vi "Main.vi"(8 "error in":errorcluster, 11 "Maestro Data Logg in":refnum<class "Maestro Data Logg.lvclass">) -> (0 "error out":errorcluster, 3 "Maestro Data Logg out":refnum<class "Maestro Data Logg.lvclass">)   [LabVIEW 2021, in "Maestro Data Logg.lvclass"]
doc: "The Queued Message Handler of a Worker."
uses:
  Maestro Data Logg.lvclass
  C:/Program Files (x86)/National Instruments/LabVIEW 2021/vi.lib/addons/_Workers/Library/Classes/Worker/Worker.lvclass
  Logging State.ctl
  Initialization Data.ctl
  <vilib>/addons/_Workers/Library/Classes/Message Queue/Message Queue.lvclass
  Maestro Data Logg.lvclass/Maestro Data Logg.ctl
  <vilib>/addons/_Workers/Library/Classes/Message/Enqueue Message to Self v2.vi
  <vilib>/addons/_Workers/Library/Classes/Message/Enqueue Message to Queue.vi
  <vilib>/addons/_Workers/Library/Classes/Message/Message.lvclass
  Maestro Control/Maestro Control.lvclass
  C:/Program Files (x86)/National Instruments/LabVIEW 2021/vi.lib/addons/_Workers/Library/Classes/Workers Object/Workers Object.lvclass
  C:/Users/flepetit/Desktop/Gentec-maestro-Labview/Workers/Maestro Data Logg/Maestro Data Logg.lvclass
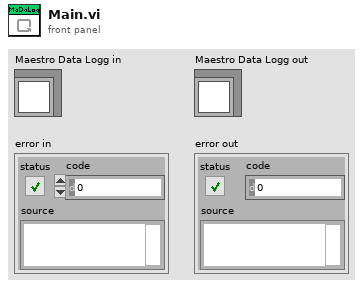
[diagram p1: front panel]
types:
  T1 = typedef "Maestro Data Logg.lvclass/Initialization Data.ctl" = cluster{"String":string, "Data Queue":refnum<queue>, "Data Notifier":refnum<notifier>, "Maestro Ctrl Queue":refnum<class "Message Queue.lvclass">, "Log File Base Path":path, "Activer les Stats":bool}
  T2 = typedef "Maestro Data Logg.lvclass/Logging State.ctl" = enum16{"Idle", "Logging"}
  T3 = enum16{"open", "open or create", "create or replace", "create", "open (read-only)"}
  T4 = cluster{"Tps(s)":dbl[], "Puiss.":dbl, "Waveform":waveform(dbl)[]}
  T5 = typedef "Workers.lvlib/Case Label.ctl" = string
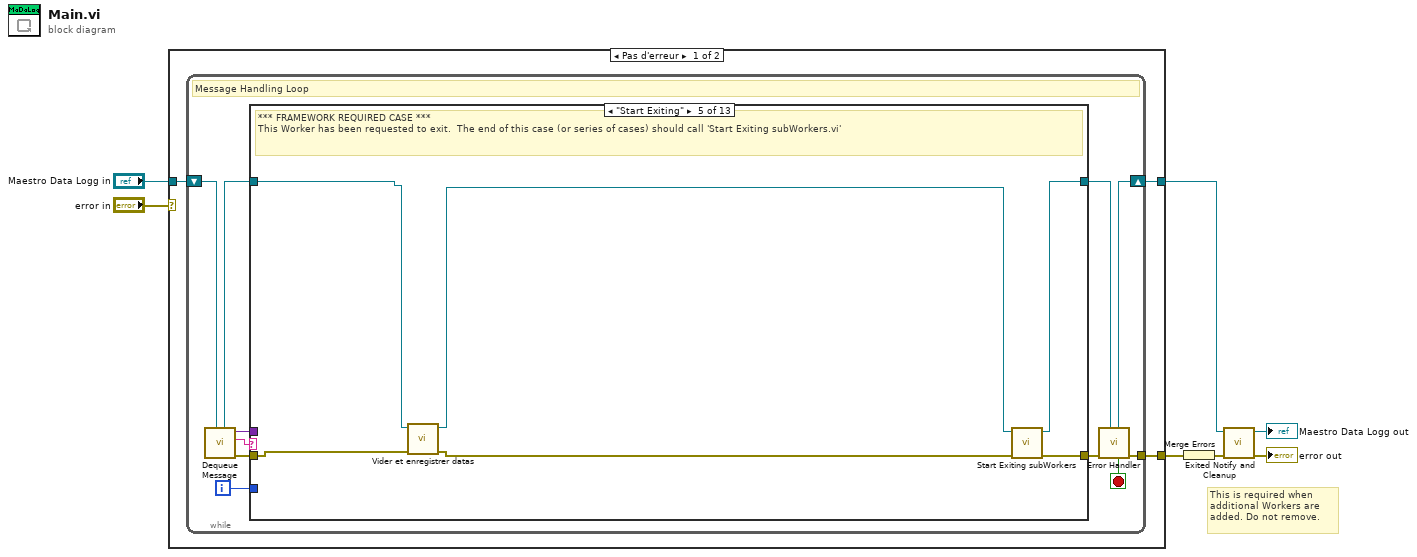
[diagram p0: block diagram]
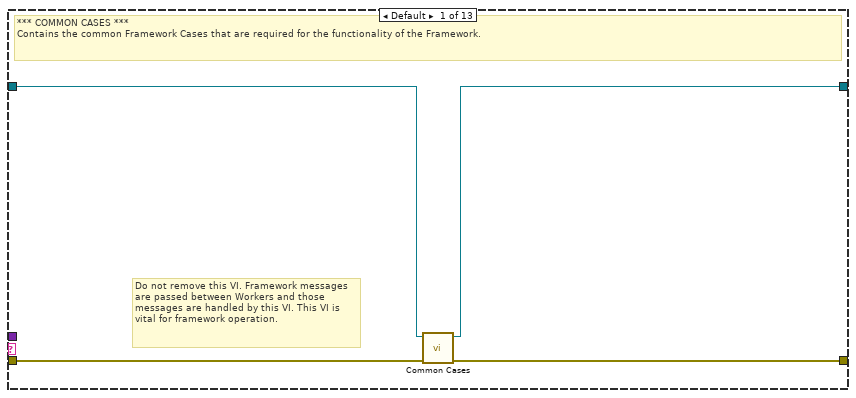
[diagram p2: hidden frame]
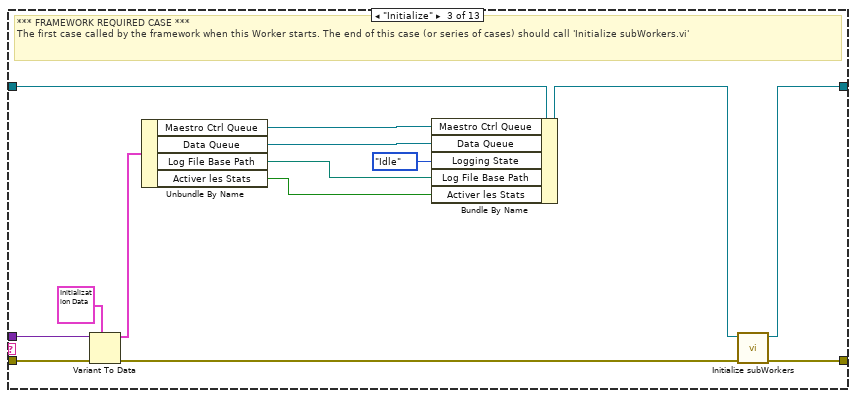
[diagram p4: hidden frame]
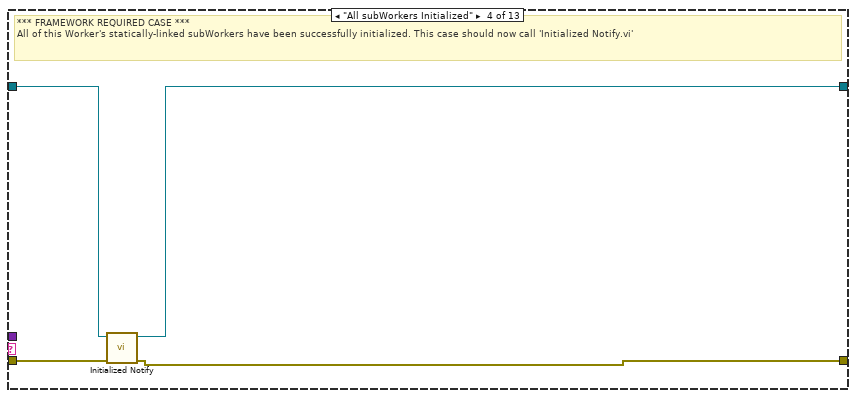
[diagram p5: hidden frame]
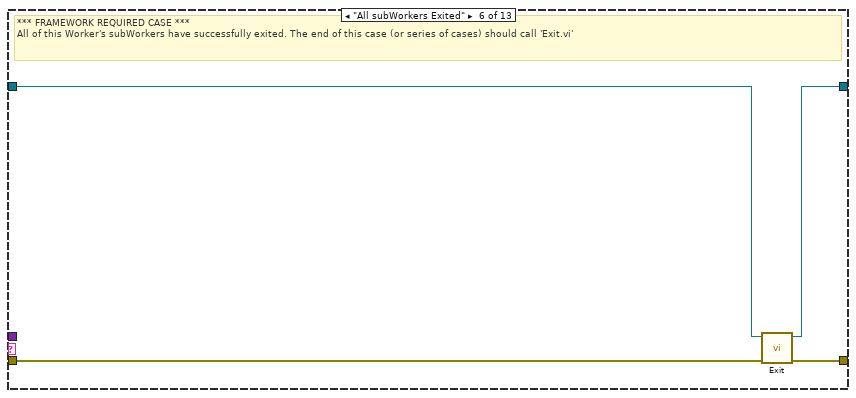
[diagram p6: hidden frame]
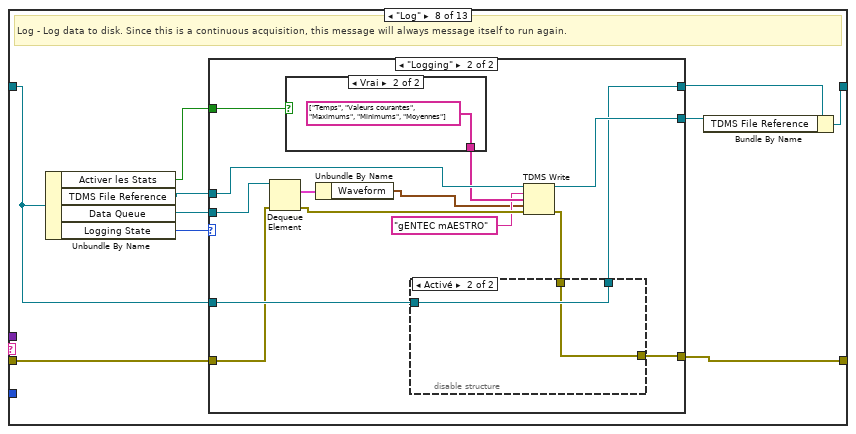
[diagram p8: hidden frame]
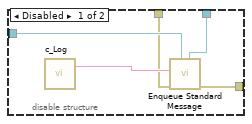
[diagram p10: hidden frame]
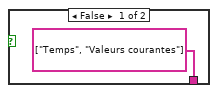
[diagram p11: hidden frame]
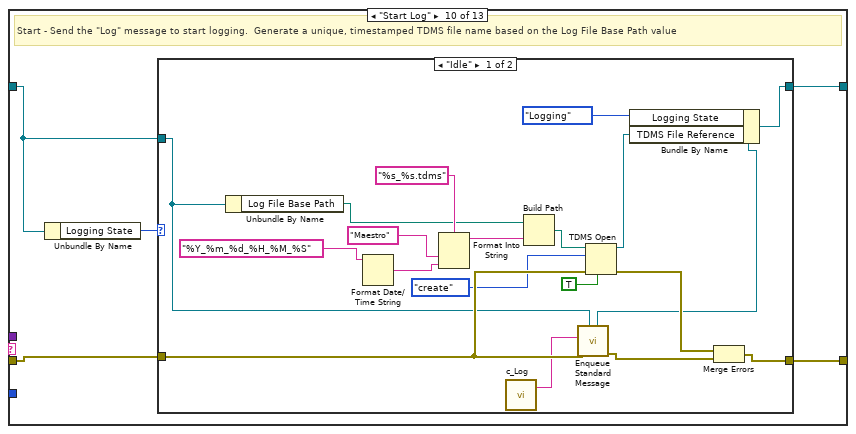
[diagram p13: hidden frame]
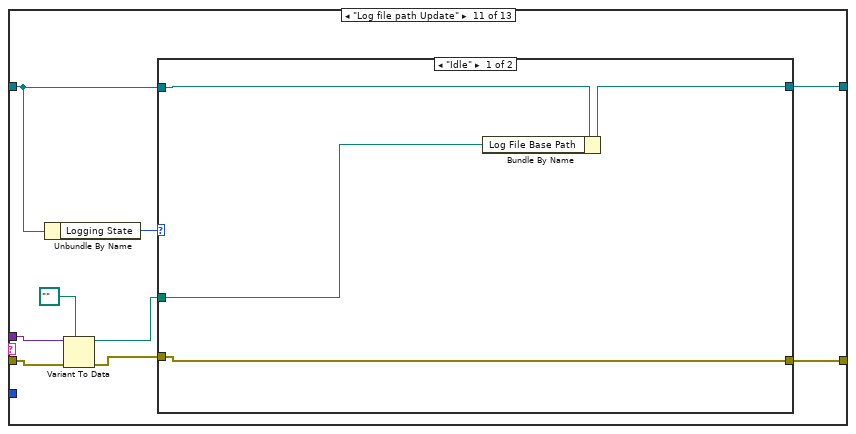
[diagram p15: hidden frame]
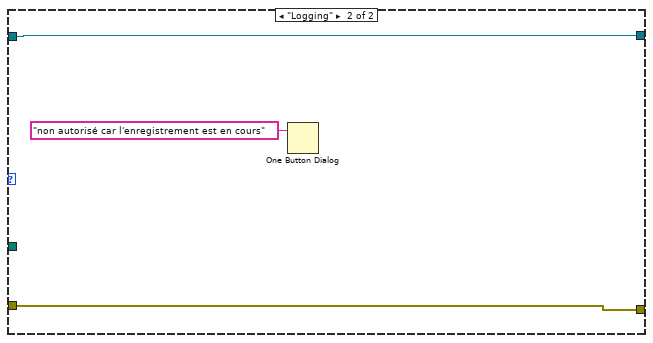
[diagram p16: hidden frame]
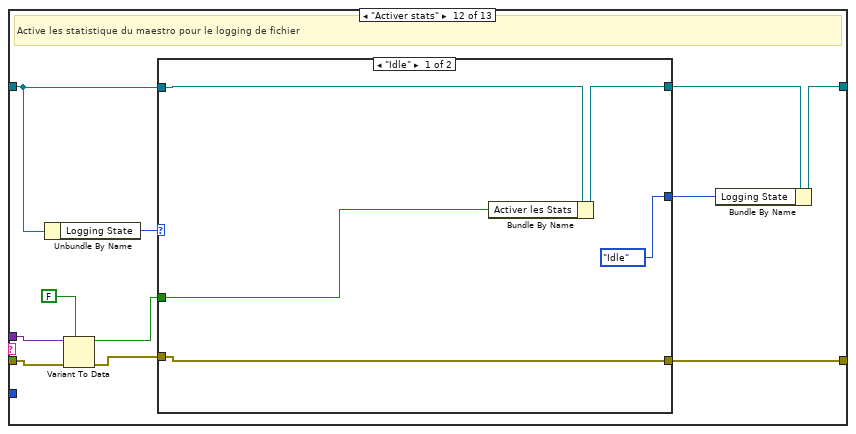
[diagram p17: hidden frame]
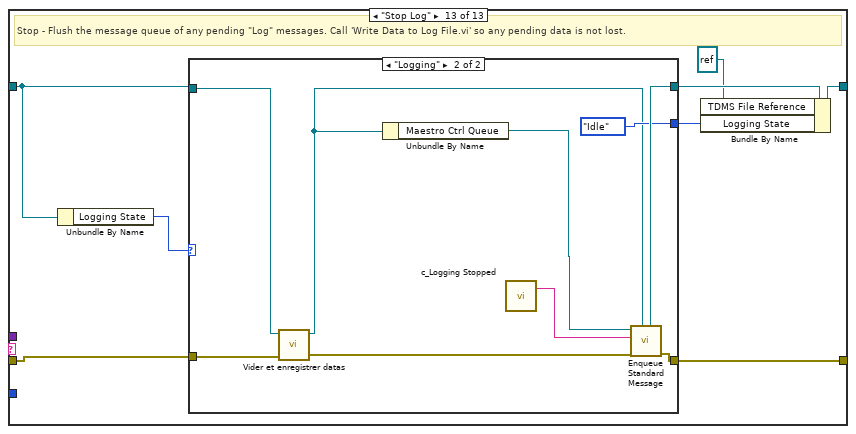
[diagram p19: hidden frame]
diagram:
  # "This is required when additional Workers are added. Do not remove."
  n1 = case shown="Pas d'erreur" "error in" {
    tunnel: "Maestro Data Logg in" -> [w8 w178]
    tunnel: [w10 w179] -> w6
    tunnel: [w9 w177] -> w7
    selector: "error in" -> [_ w180]
    frame No Error {
      n2 = while {
        shift-right: [w19] -> w9
        shift-left: w8 -> [w21]
        tunnel: [w20] -> w10
        i -> [w11]
        stop <- w12 stop-if-true
        # "Message Handling Loop"
        n3 = call-dynamic "Dequeue Message.vi"("Worker"=w21) -> ("error out"=w18:errorcluster, "Case out"=w13:string, "Data out"=w14:variant, "Worker out"=w16:refnum<class "Maestro Data Logg.lvclass">)  [unwired: 6 in, 1 out]
        n4 = case "Worker MHL Case Structure (DO NOT CHANGE LABEL NAME)" shown="\"Start Exiting\"" w13 {
          tunnel: w18 -> [w25 w26 w39 w45 w49 w55 w56 w66 w94 w96 w126 w144 w161]
          tunnel: [w24 w26 w41 w43 w51 w54 w56 w59 w94 w97 w127 w145 w162] -> w17
          tunnel: w16 -> [w23 w27 w36 w44 w47 w53 w57 w65 w95 w99 w129 w147 w163]
          tunnel: [w22 w27 w40 w42 w50 w52 w57 w60 w95 w98 w128 w139 w159] -> w15
          tunnel: w14 -> [_ _ w37 _ _ _ _ _ _ _ w124 w142 _]
          tunnel: w11 -> [_ _ _ _ _ _ _ _ _ _ _ _ _]
          frame Default {
            # "Do not remove this VI. Framework messages are passed between Workers and those messages are handled by this VI. This VI is vital for framework operation."
            # "*** COMMON CASES ***\nContains the common Framework Cases that are required for the functionality of the Framework."
            n5 = call-dynamic "Common Cases.vi"("error in"=w25, "Worker in"=w23) -> ("error out"=w24:errorcluster, "Worker out"=w22:refnum<class "Maestro Data Logg.lvclass">)  [unwired: 8 in]
          }
          frame "------ FRAMEWORK REQUIRED CASES ------" {
            # "Start of Framework Required Cases"
          }
          frame "Initialize" {
            # "*** FRAMEWORK REQUIRED CASE ***\nThe first case called by the framework when this Worker starts. The end of this case (or series of cases) should call 'Initialize subWorkers.vi'"
            n6 = Variant To Data(error in=w39, type=T1 {"String"="", "Data Queue"=refnum, "Data Notifier"=refnum, "Maestro Ctrl Queue"=refnum, "Log File Base Path"=path "", "Activer les Stats"=FALSE} ("Cluster"), Variant=w37) -> (data=w35:T1, error out=w38:errorcluster)
            n7 = Unbundle By Name(w35) -> ("Maestro Ctrl Queue"=w33:refnum<class "Message Queue.lvclass">, "Data Queue"=w32:refnum<queue>, "Log File Base Path"=w30:path, "Activer les Stats"=w29:bool)
            n8 = Bundle By Name(cluster=w36, "Maestro Ctrl Queue"=w33, "Data Queue"=w32, "Logging State"=Logging_State."Idle", "Log File Base Path"=w30, "Activer les Stats"=w29) -> (w34:refnum<class "Maestro Data Logg.lvclass">)
            n9 = call-dynamic "Initialize subWorkers.vi"("error in"=w38, "Worker"=w34) -> ("error out"=w41:errorcluster, "dup Worker out"=w40:refnum<class "Maestro Data Logg.lvclass">)  [unwired: 8 in]
          }
          frame "All subWorkers Initialized" {
            # "*** FRAMEWORK REQUIRED CASE ***\nAll of this Worker's statically-linked subWorkers have been successfully initialized. This case should now call 'Initialized Notify.vi'"
            n10 = call-dynamic "Initialized Notify.vi"("error in"=w45, "Worker"=w44) -> ("error out"=w43:errorcluster, "dup Worker out"=w42:refnum<class "Maestro Data Logg.lvclass">)  [unwired: 8 in]
          }
          frame "Start Exiting" {
            # "*** FRAMEWORK REQUIRED CASE ***\nThis Worker has been requested to exit.  The end of this case (or series of cases) should call 'Start Exiting subWorkers.vi'"
            n11 = call "Vider et enregistrer datas.vi"("error in (no error)"=w49, "Maestro Data Logg en entrée"=w47) -> ("error out"=w48:errorcluster, "Maestro Data Logg en sortie"=w46:refnum<class "Maestro Data Logg.lvclass">)  [unwired: 8 in]
            n12 = call-dynamic "Start Exiting subWorkers.vi"("error_in"=w48, "Worker"=w46) -> ("error out"=w51:errorcluster, "dup Worker out"=w50:refnum<class "Maestro Data Logg.lvclass">)  [unwired: 8 in]
          }
          frame "All subWorkers Exited" {
            # "*** FRAMEWORK REQUIRED CASE ***\nAll of this Worker's subWorkers have successfully exited. The end of this case (or series of cases) should call 'Exit.vi'"
            n13 = call-dynamic "Exit.vi"("error_in"=w55, "Worker"=w53) -> ("error out"=w54:errorcluster, "dup Worker out"=w52:refnum<class "Maestro Data Logg.lvclass">)  [unwired: 8 in]
          }
          frame "------------------Himself-------------------------" {
            # "End of Framework Required Cases"
          }
          frame "Log" {
            # "Log - Log data to disk. Since this is a continuous acquisition, this message will always message itself to run again."
            n14 = Unbundle By Name(w65) -> ("Activer les Stats"=w58:bool, "TDMS File Reference"=w63:refnum<k34>, "Data Queue"=w64:refnum<queue>, "Logging State"=w67:T2)
            n15 = case shown="\"Logging\"" w67 {
              tunnel: [w70 w74] -> w61
              tunnel: w66 -> [w69 w79]
              tunnel: [w69 w72] -> w59
              tunnel: w65 -> [w70 w84]
              tunnel: w64 -> [_ w82]
              tunnel: w63 -> [w68 w80]
              tunnel: [w68 w75] -> w62
              tunnel: w58 -> [_ w71]
              frame "Idle" {
              }
              frame "Logging" {
                n16 = Dequeue Element(queue=w82, error in (no error)=w79) -> (element=w81:T4, error out=w83:errorcluster)  [unwired: 1 in, 2 out]
                n17 = case shown="Vrai" w71 {
                  tunnel: [string[] ["Temps", "Valeurs courantes"] ("nom des voies en entrée (Sans titre)") string[] ["Temps", "Valeurs courantes", "Maximums", "Minimums", "Moyennes"] ("nom des voies en entrée (Sans titre)")] -> w78
                  frame False {
                  }
                  frame True {
                  }
                }
                n18 = Unbundle By Name(w81) -> ("Waveform"=w76:waveform(dbl)[])
                n19 = TDMS Write(0:w80, 5:"gENTEC mAESTRO" ("nom du groupe en entrée (Sans titre)"), 7:w78, 9:w76, 11:w83) -> (4:w75:refnum<k34>, 15:w73:errorcluster)  [unwired: 1 in, 2 out]
                n20 = disable-structure shown="Activé" {
                  disable-tunnel: w84 -> [w89 w91]
                  disable-tunnel: [w87 w91] -> w74
                  disable-tunnel: w73 -> [w86 w90]
                  disable-tunnel: [w85 w90] -> w72
                  frame Disabled {
                    n21 = call "c_Log.vi"() -> ("Case Label"=w88:T5)  [unwired: 1 in]
                    n22 = call-poly <vilib>:"Enqueue Standard Message.vi"("Worker"=w89, "error in"=w86, "Case Label"=w88) -> ("error out"=w85:errorcluster, "dup Worker out"=w87:refnum<class "Maestro Data Logg.lvclass">)  [unwired: 7 in]
                  }
                  frame Enabled {
                  }
                }
              }
            }
            n23 = Bundle By Name(cluster=w61, "TDMS File Reference"=w62) -> (w60:refnum<class "Maestro Data Logg.lvclass">)
          }
          frame "------------From Maestro Control--------------" {
            # "End of Framework Required Cases"
          }
          frame "Start Log" {
            # "Start - Send the \"Log\" message to start logging.  Generate a unique, timestamped TDMS file name based on the Log File Base Path value"
            n24 = Unbundle By Name(w99) -> ("Logging State"=w100:T2)
            n25 = case shown="\"Idle\"" w100 {
              tunnel: w99 -> [w108 w121]
              tunnel: [w109 w121] -> w98
              tunnel: [w115 w120] -> w97
              tunnel: w96 -> [w117 w120]
              frame "Idle" {
                n26 = Unbundle By Name(w108) -> ("Log File Base Path"=w104:path)
                n27 = Format Date/Time String(time format string (%c)="%Y_%m_%d_%H_%M_%S") -> (date/time string=w105:string)  [unwired: 2 in]
                n28 = Format Into String(format string="%s_%s.tdms", "Maestro" ("entrée 1"), w105) -> (resulting string=w119:string)  [unwired: 2 in, 1 out]
                n29 = call "c_Log.vi"() -> ("Case Label"=w101:T5)  [unwired: 1 in]
                n30 = Build Path(base path=w104, name or relative path=w119) -> (appended path=w113:path)
                n31 = call-poly <vilib>:"Enqueue Standard Message.vi"("Worker"=w108, "error in"=w117, "Case Label"=w101) -> ("error out"=w116:errorcluster, "dup Worker out"=w107:refnum<class "Maestro Data Logg.lvclass">)  [unwired: 7 in]
                n32 = TDMS Open(6:TRUE ("désactiver la bufférisation ? (V)"), 8:w117, 10:T3."create" ("operation (0:open)"), 11:w113) -> (0:w114:errorcluster, 3:w110:refnum<k34>)  [unwired: 3 in]
                n33 = Bundle By Name(cluster=w107, "Logging State"=Logging_State."Logging", "TDMS File Reference"=w110) -> (w109:refnum<class "Maestro Data Logg.lvclass">)
                n34 = Merge Errors(w114, w116) -> (w115:errorcluster)
              }
              frame "Logging" {
              }
            }
          }
          frame "Log file path Update" {
            n35 = Unbundle By Name(w129) -> ("Logging State"=w130:T2)
            n36 = Variant To Data(error in=w126, type=path "", Variant=w124) -> (data=w122:path, error out=w125:errorcluster)
            n37 = case shown="\"Idle\"" w130 {
              tunnel: w129 -> [w134 w137]
              tunnel: [w133 w137] -> w128
              tunnel: [w131 w136] -> w127
              tunnel: w125 -> [w131 w136]
              tunnel: w122 -> [w132 _]
              frame "Idle" {
                n38 = Bundle By Name(cluster=w134, "Log File Base Path"=w132) -> (w133:refnum<class "Maestro Data Logg.lvclass">)
              }
              frame "Logging" {
                n39 = One Button Dialog(message="non autorisé car l'enregistrement est en cours") -> ()  [unwired: 1 in, 1 out]
              }
            }
          }
          frame "Activer stats" {
            # "Active les statistique du maestro pour le logging de fichier"
            n40 = Unbundle By Name(w147) -> ("Logging State"=w148:T2)
            n41 = Variant To Data(error in=w144, type=FALSE, Variant=w142) -> (data=w140:bool, error out=w143:errorcluster)
            n42 = case shown="\"Idle\"" w148 {
              selector: w148 -> [_ w154]
              tunnel: w147 -> [w153 w156]
              tunnel: [w152 w156] -> w146
              tunnel: [w150 w155] -> w145
              tunnel: w143 -> [w150 w155]
              tunnel: w140 -> [w151 _]
              tunnel: [Logging_State."Idle" ("Logging State") w154] -> w138
              frame "Idle" {
                n43 = Bundle By Name(cluster=w153, "Activer les Stats"=w151) -> (w152:refnum<class "Maestro Data Logg.lvclass">)
              }
              frame "Logging" {
              }
            }
            n44 = Bundle By Name(cluster=w146, "Logging State"=w138) -> (w139:refnum<class "Maestro Data Logg.lvclass">)
          }
          frame "Stop Log" {
            # "Stop - Flush the message queue of any pending \"Log\" messages. Call 'Write Data to Log File.vi' so any pending data is not lost."
            n45 = Unbundle By Name(w163) -> ("Logging State"=w164:T2)
            n46 = case shown="\"Logging\"" w164 {
              selector: w164 -> [w165 _]
              tunnel: w163 -> [w166 w171]
              tunnel: [w166 w174] -> w160
              tunnel: [w167 w176] -> w162
              tunnel: w161 -> [w167 w169]
              tunnel: [w165 Logging_State."Idle" ("Logging State")] -> w157
              frame "Idle" {
              }
              frame "Logging" {
                n47 = call "Vider et enregistrer datas.vi"("error in (no error)"=w169, "Maestro Data Logg en entrée"=w171) -> ("error out"=w168:errorcluster, "Maestro Data Logg en sortie"=w170:refnum<class "Maestro Data Logg.lvclass">)  [unwired: 8 in]
                n48 = Unbundle By Name(w170) -> ("Maestro Ctrl Queue"=w175:refnum<class "Message Queue.lvclass">)
                n49 = call "c_Logging Stopped.vi"() -> ("Case Label"=w173:T5)  [unwired: 1 in]
                n50 = call-poly <vilib>:"Enqueue Standard Message.vi"("Worker"=w170, "error in"=w168, "Case Label"=w173, "Message Queue"=w175) -> ("error out"=w176:errorcluster, "dup Worker out"=w174:refnum<class "Maestro Data Logg.lvclass">)  [unwired: 5 in, 1 out]
              }
            }
            n51 = Bundle By Name(cluster=w160, "TDMS File Reference"=refnum<k34> refnum ("Logging Configuration.TDMS File Reference"), "Logging State"=w157) -> (w159:refnum<class "Maestro Data Logg.lvclass">)
          }
        }
        n52 = call-dynamic "Error Handler.vi"("Worker"=w15, "error_in"=w17) -> ("error out"=w20:errorcluster, "Stop Loop"=w12:bool, "Worker out"=w19:refnum<class "Maestro Data Logg.lvclass">)  [unwired: 7 in]
      }
    }
    frame Error {
      n53 = call-dynamic "Error Handler.vi"("Worker"=w178, "error_in"=w180) -> ("error out"=w179:errorcluster, "Worker out"=w177:refnum<class "Maestro Data Logg.lvclass">)  [unwired: 7 in, 1 out]
    }
  }
  n54 = Merge Errors(w6) -> (w3:errorcluster)
  n55 = call-dynamic "Exited Notify and Cleanup.vi"("error_in"=w3, "Worker"=w7) -> ("error out"=→"error out":errorcluster, "dup Worker out"=→"Maestro Data Logg out":refnum<class "Maestro Data Logg.lvclass">)  [unwired: 8 in]
